vi "Add Instrument.vi"(8 "error in":errorcluster, 10 "Instrument":refnum<class "Instrument.lvclass">, 11 "Host Measure and Stimulus Subsystems in":refnum<class "Host Measure and Stimulus Subsystems.lvclass">) -> (0 "error out":errorcluster, 3 "Host Measure and Stimulus Subsystems out":refnum<class "Host Measure and Stimulus Subsystems.lvclass">)   [LabVIEW 2023, in "HAL GOOP4.lvlib" / "Host Measure and Stimulus Subsystems.lvclass"]
uses:
  Host Measure and Stimulus Subsystems.lvclass
  Host Measure and Stimulus Subsystems.lvclass/Host Measure and Stimulus Subsystems.ctl
  <vilib>/Utility/miscctls.llb/LVMapReplaceAction.ctl
  <vilib>/Utility/error.llb/Error Cluster From Error Code.vi
  <vilib>/ErrorRing/Error Ring.xnode
  Instrument/Instrument.lvclass
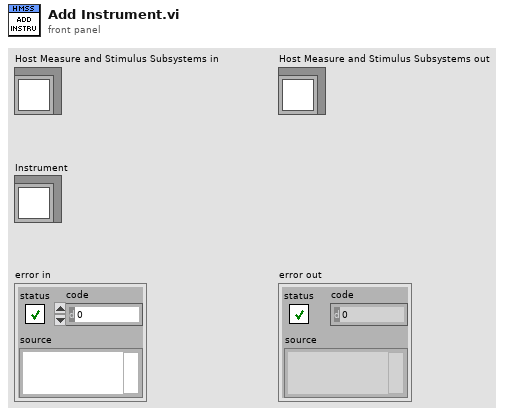
[diagram p1: front panel]
types:
  T1 = map{string, cluster{"Instrument":refnum<class "Instrument.lvclass">, "Ref Count":u8}}
  T2 = typedef "LVMapReplaceAction.ctl" = enum32{"Modify Entry only if found", "Add or Modify Entry", "Delete Entry"}
  T3 = cluster{"Instrument":refnum<class "Instrument.lvclass">, "Ref Count":u8}
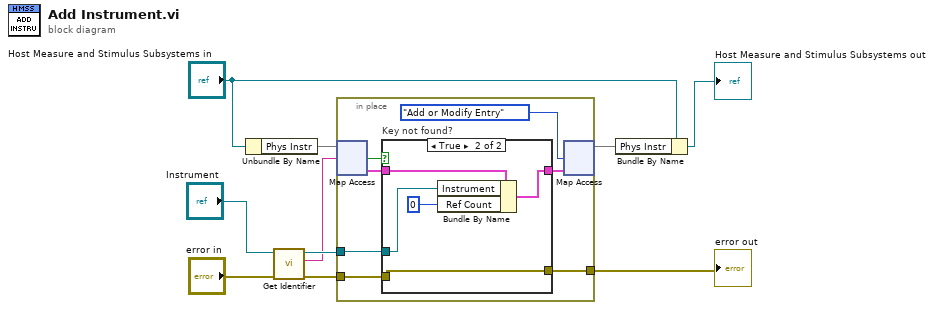
[diagram p0: block diagram]
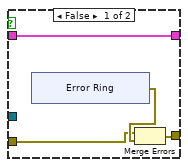
[diagram p2: hidden frame]
diagram:
  n1 = Unbundle By Name("Host Measure and Stimulus Subsystems in") -> ("Phys Instr"=w8:T1)
  n2 = call "Get Identifier.vi"("Error In"="error in", "reference in"="Instrument") -> ("Error Out"=w5:errorcluster, "Instr Name"=w6:string, "reference out"=w7:refnum<class "Instrument.lvclass">)  [unwired: 7 in]
  n3 = in-place {
    in-place-border: w7 -> [w15]
    in-place-border: w5 -> [w12]
    in-place-border: [w11] -> w2
    n4 = in-place-map #1(w8, w6) -> (w16:T3, w17:bool)  [unwired: 1 in]
    n5 = case "Key not found?" shown="True" w17 {
      tunnel: w16 -> [w18 w28]
      tunnel: [w18 w30] -> w13
      tunnel: w15 -> [_ w31]
      tunnel: w12 -> [w20 w29]
      tunnel: [w19 w29] -> w11
      frame False {
        n6 = xnode "Error Ring"() -> ("error out"=w21:errorcluster)
        n7 = Merge Errors(w20, w21) -> (w19:errorcluster)
      }
      frame True {
        n8 = Bundle By Name(cluster=w28, "Instrument"=w31, "Ref Count"=u8 0) -> (w30:T3)
      }
    }
    n9 = in-place-map #1(w13, LVMapReplaceAction."Add or Modify Entry" ("action")) -> (w9:T1)  [unwired: 2 out]
  }
  "error out" <- w2
  n10 = Bundle By Name(cluster="Host Measure and Stimulus Subsystems in", "Phys Instr"=w9) -> (→"Host Measure and Stimulus Subsystems out":refnum<class "Host Measure and Stimulus Subsystems.lvclass">)
